vi "Write_Read_TXT.vi"(6 "Read/Write":enum16{"Read", "Write"}(ring), 7 "String":string, 8 "error in (no error)":errorcluster, 9 "access (0:read/write)":enum16{"read/write", "read-only", "write-only"}(ring), 10 "operation (0:open)":T1(ring), 11 "file path (dialog if empty)":path) -> (0 "error out":errorcluster, 3 "TXT":string)   [LabVIEW 2013]
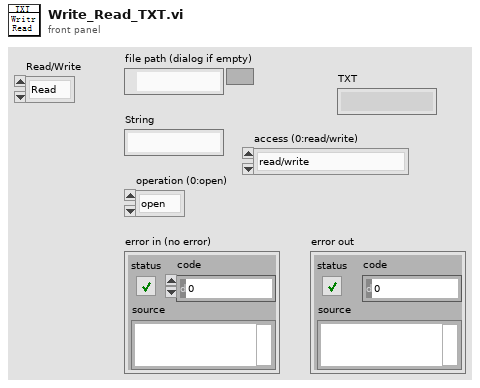
[diagram p1: front panel]
types:
  T1 = enum16{"open", "replace", "create", "open or create", "replace or create", "replace or create with confirmation"}
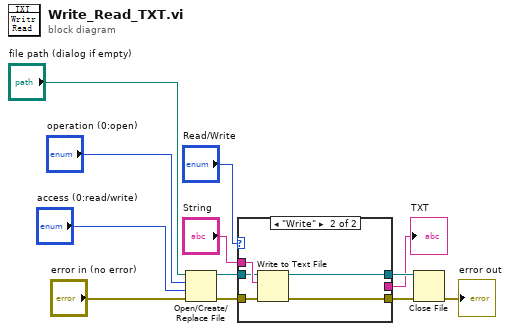
[diagram p0: block diagram]
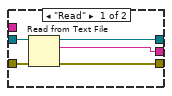
[diagram p2: hidden frame]
diagram:
  n1 = Open/Create/Replace File(file path (use dialog)="file path (dialog if empty)", error in="error in (no error)", operation (0:open)="operation (0:open)", access (0:read/write)="access (0:read/write)") -> (refnum out=w4:refnum<file>, error out=w8:errorcluster)  [unwired: 2 in, 1 out]
  n2 = case shown="\"Write\"" "Read/Write" {
    tunnel: "String" -> [_ w22]
    tunnel: w8 -> [w17 w21]
    tunnel: [w16 w20] -> w7
    tunnel: [w14 w19] -> w6
    tunnel: w4 -> [w15 w18]
    tunnel: [w13 _] -> w2
    frame "Read" {
      n3 = Read from Text File(file (use dialog)=w15, error in=w17) -> (refnum out=w14:refnum<file>, text=w13:string, error out=w16:errorcluster)  [unwired: 2 in, 1 out]
    }
    frame "Write" {
      n4 = Write to Text File(file (use dialog)=w18, text=w22, error in=w21) -> (refnum out=w19:refnum<file>, error out=w20:errorcluster)  [unwired: 1 in, 1 out]
    }
  }
  "TXT" <- w2
  n5 = Close File(refnum=w6, error in=w7) -> (error out=→"error out":errorcluster)  [unwired: 1 out]
